vi "MoveArmToHigh10Ft.vi"   [LabVIEW 2019]
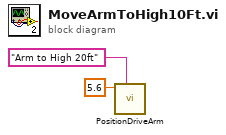
[diagram p0: block diagram]
diagram:
  n1 = call "PositionDriveArm.vi"("Description"="Arm to High 20ft", "Position"=5.6) -> ()  [unwired: 9 in, 1 out]
